vi "MH_DeInitDone.vi"(8 "error in (no error)":errorcluster, 11 "SinglePhotonInterferenceUI in":refnum<class "SinglePhotonInterferenceUI.lvclass">) -> (0 "error out":errorcluster, 3 "SinglePhotonInterferenceUI out":refnum<class "SinglePhotonInterferenceUI.lvclass">)   [LabVIEW 2023, in "SinglePhotonInterferenceUI.lvlib" / "SinglePhotonInterferenceUI.lvclass"]
uses:
  SinglePhotonInterferenceUI.lvclass
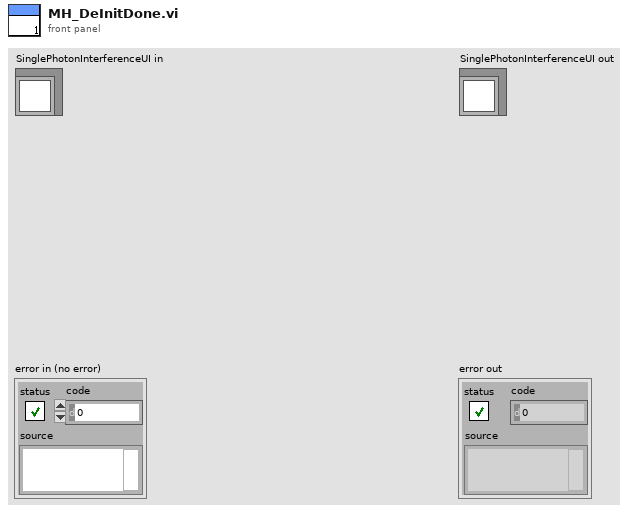
[diagram p1: front panel]
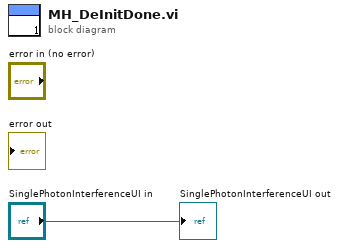
[diagram p0: block diagram]
diagram:
  "SinglePhotonInterferenceUI out" <- "SinglePhotonInterferenceUI in"
